vi "getOffsetToUTC.vi"(11 "Epoch (GPS)":refnum<class "Epoch.GPS.lvclass">) -> (2 "Offset to UTC":i64)   [LabVIEW 2013, in "Epoch.GPS.lvclass"]
uses:
  Epoch.GPS.lvclass
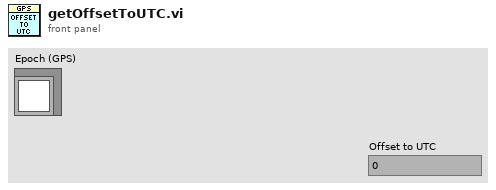
[diagram p1: front panel]
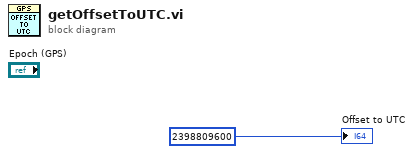
[diagram p0: block diagram]
diagram:
  "Offset to UTC" <- i64 2398809600 ("Timestamp Offset")
